vi "Rozbicie tekstu na współrzędną w formacie D.vi"(0 "Współrzędna tekstowa":string) -> (2 "Druga współrzędna":string, 3 "D":dbl, 6 "Kierunek":string)   [LabVIEW 2015, in "Biblioteka moduł map v3.lvlib" / "Konwersja wsp.lvlib" / "Wyciągnięcie z tekstu współrzędnej.lvlib"]
doc: "SubVI odfiltrowuje wartość stopni pierwszej napotkanej współrzędnej oraz jej kierunek. Dodatkowo otrzyjmujemy dalszą część tekstu, która odpowiada współrzędnej drugiej (nieodfiltrowanej jeszcze)."
uses:
  <vilib>/regexp/Match Regular Expression.xnode
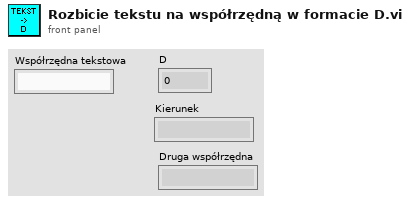
[diagram p1: front panel]
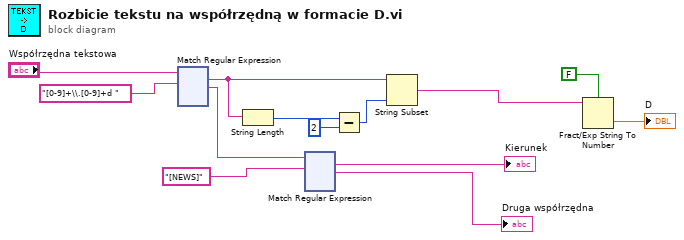
[diagram p0: block diagram]
diagram:
  n1 = xnode "Match Regular Expression"("input string"="Współrzędna tekstowa", "regular expression"="[0-9]+\\.[0-9]+d ") -> ("whole match"=w9:string, "after match"=w5:string)  [unwired: 4 in, 3 out]
  n2 = String Length(string=w9) -> (length=w11:i32)
  n3 = xnode "Match Regular Expression"("input string"=w5, "regular expression"="[NEWS]") -> ("whole match"=→"Kierunek":string, "after match"=→"Druga współrzędna":string)  [unwired: 4 in, 3 out]
  n4 = Subtract(x=w11, y=2) -> (x-y=w13:i32)
  n5 = String Subset(string=w9, length (rest)=w13) -> (substring=w7:string)  [unwired: 1 in]
  n6 = Fract/Exp String To Number(use system decimal point (T)=FALSE, string=w7) -> (number=→"D":dbl)  [unwired: 2 in, 1 out]
